vi "New.vi"(11 "VoltageMeasArray":dbl[](array[numeric])) -> (3 "VoltageResult.lvclass":refnum<class "VoltageResult.lvclass">)   [LabVIEW 2020, in "VoltageResult.lvclass"]
uses:
  VoltageResult.lvclass
  VoltageResult.lvclass/VoltageResult.ctl
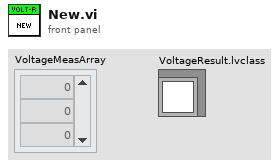
[diagram p1: front panel]
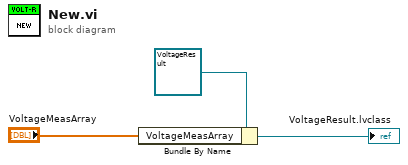
[diagram p0: block diagram]
diagram:
  n1 = Bundle By Name(cluster=refnum<class "VoltageResult.lvclass"> refnum ("VoltageResult.lvclass"), "VoltageMeasArray"="VoltageMeasArray") -> (→"VoltageResult.lvclass":refnum<class "VoltageResult.lvclass">)
